vi "logic.vi"(7 "transition_queue":refnum<queue>, 8 "error in (no error)":errorcluster, 11 "data_in":T1) -> (0 "error out":errorcluster, 1 "data out":variant, 2 "change":bool, 3 "data_out":T1)   [LabVIEW 2015, in "lv-recipe-machine.lvlib"]
uses:
  lv-recipe-machine.lvlib
  _controls/recipe_data.ctl
  public/_controls/mode.ctl
  public/_controls/manual_state.ctl
  public/_controls/automatic_state.ctl
  _controls/timer.ctl
  public/_controls/recipe_step.ctl
  public/_controls/transition.ctl
  _controls/timers.ctl
  public/_controls/error.ctl
  _controls/timer_command.ctl
  _controls/automatic_vi_variant_data.ctl
  <vilib>/ptbypt/NI_PtbyPt.lvlib
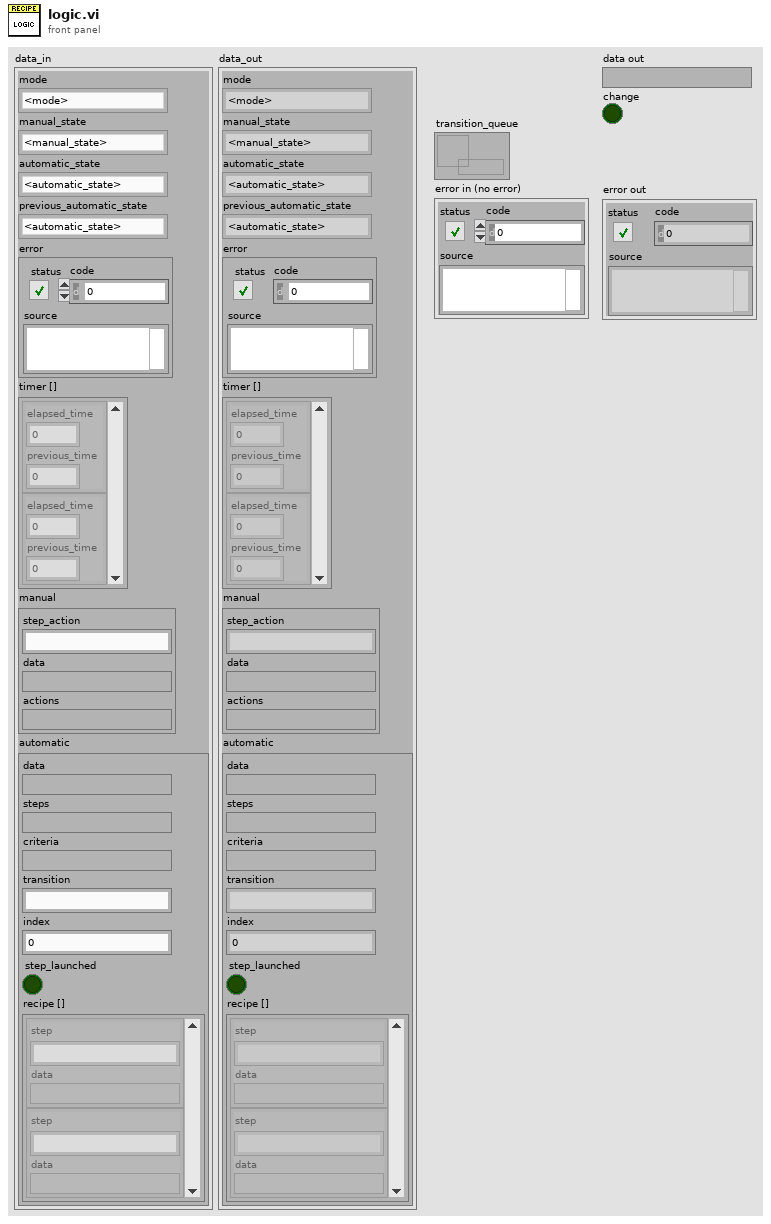
[diagram p1: front panel]
types:
  T1 = typedef "lv-recipe-machine.lvlib/recipe_data.ctl" = cluster{"mode":T2, "manual_state":T3, "automatic_state":T4, "previous_automatic_state":T4, "error":errorcluster, "timer []":T5[], "manual":cluster{"step_action":string, "data":variant, "actions":variant}, "automatic":cluster{"data":variant, "steps":variant, "criteria":variant, "transition":string, "index":i32, "step_launched":bool, "recipe []":T6[]}}
  T2 = typedef "lv-recipe-machine.lvlib/mode.ctl" = enum16{"<mode>", "manual", "automatic", "<null>"}
  T3 = typedef "lv-recipe-machine.lvlib/manual_state.ctl" = enum16{"<manual_state>", "failed", "action", "running", "idle", "<null>"}
  T4 = typedef "lv-recipe-machine.lvlib/automatic_state.ctl" = enum16{"<automatic_state>", "failed", "idle", "running", "paused", "stopped", "<null>"}
  T5 = typedef "lv-recipe-machine.lvlib/timer.ctl" = cluster{"elapsed_time":dbl, "previous_time":dbl}
  T6 = typedef "lv-recipe-machine.lvlib/recipe_step.ctl" = cluster{"step":string, "data":variant}
  T7 = typedef "lv-recipe-machine.lvlib/error.ctl" = enum16{"<error>", "bad_command", "command_queue_timeout", "stop_notifier_timeout", "die_command_timeout", "not_in_manual_mode", "not_in_automatic_mode", "not_in_automatic_idle", "not_in_automatic_running", "not_in_automatic_paused", "automatic_step_not_found", "manual_action_not_found", "automatic_not_transition_vi", "transition_step_not_found", "unsupported_vi_type", "manual_block_timeout", "<null>"}
  T8 = typedef "lv-recipe-machine.lvlib/timers.ctl" = enum16{"<timers>", "step", "recipe", "<null>"}
  T9 = typedef "lv-recipe-machine.lvlib/timer_command.ctl" = enum16{"<timer_command>", "initialize", "start", "read", "pause", "resume", "stop", "<null>"}
  T10 = typedef "lv-recipe-machine.lvlib/automatic_vi_variant_data.ctl" = cluster{"current_state":T4, "previous_state":T4, "criteria":variant, "data":variant, "recipe_data":variant, "index":i32, "step":string, "steps":variant}
  T11 = cluster{"data":variant, "steps":variant, "criteria":variant, "transition":string, "index":i32, "step_launched":bool, "recipe []":T6[]}
  T12 = cluster{"step_action":string, "data":variant, "actions":variant}
  T13 = typedef "lv-recipe-machine.lvlib/transition.ctl" = cluster{"next_index":i32, "data":variant, "recipe_data":variant, "error":errorcluster}
  T14 = cluster{"recipe_data out":variant, "error IO":errorcluster}
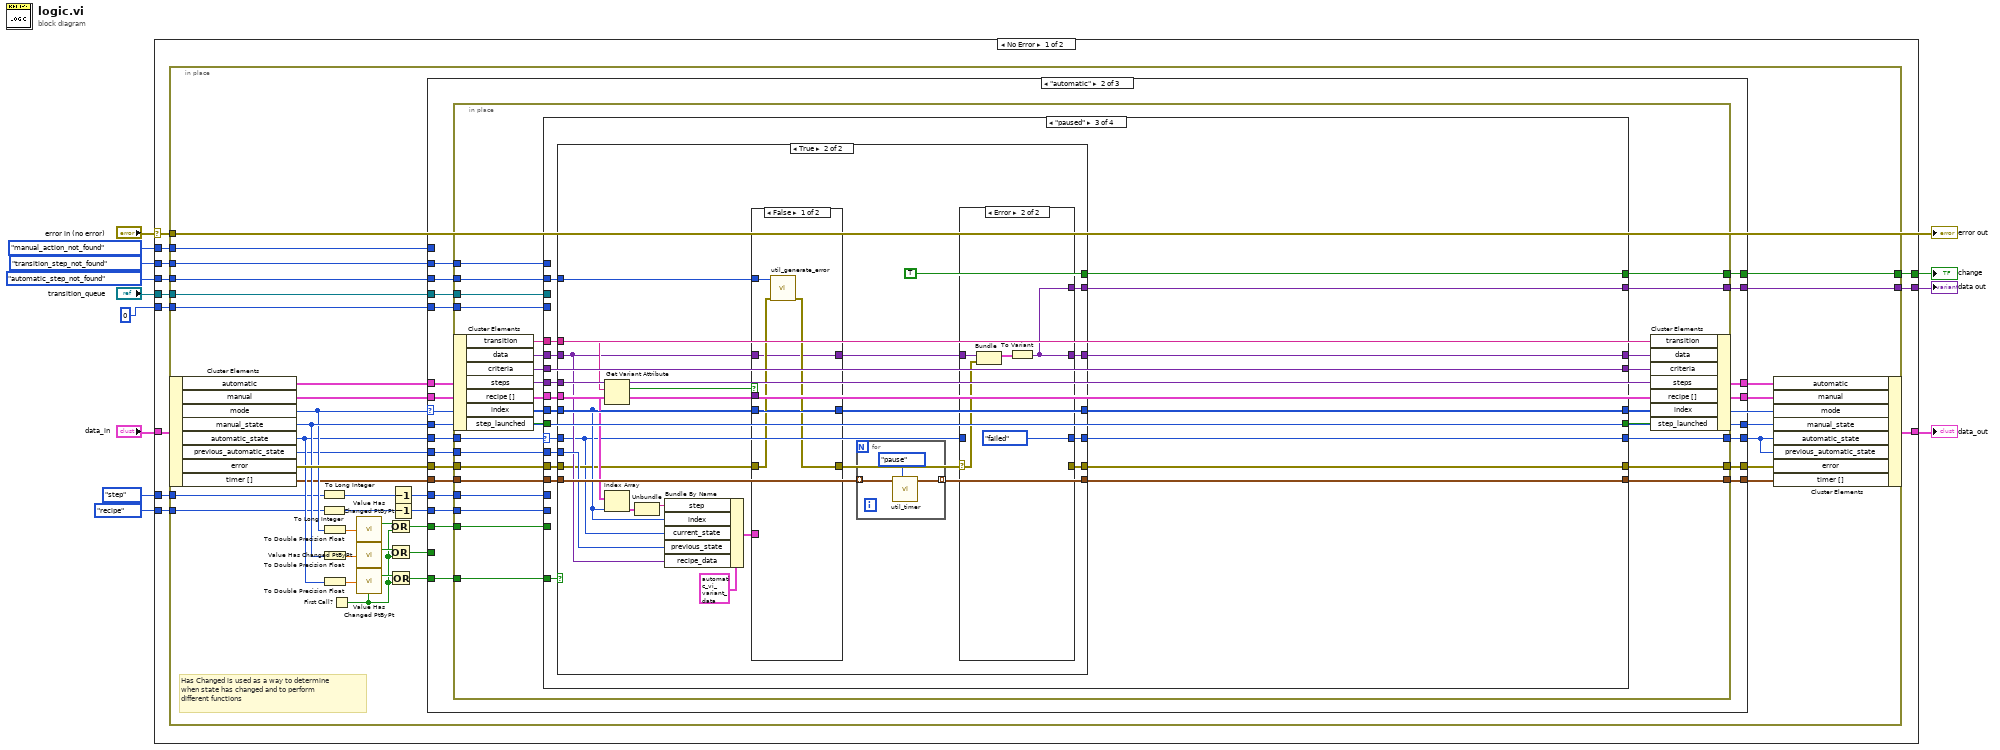
[diagram p0: block diagram]
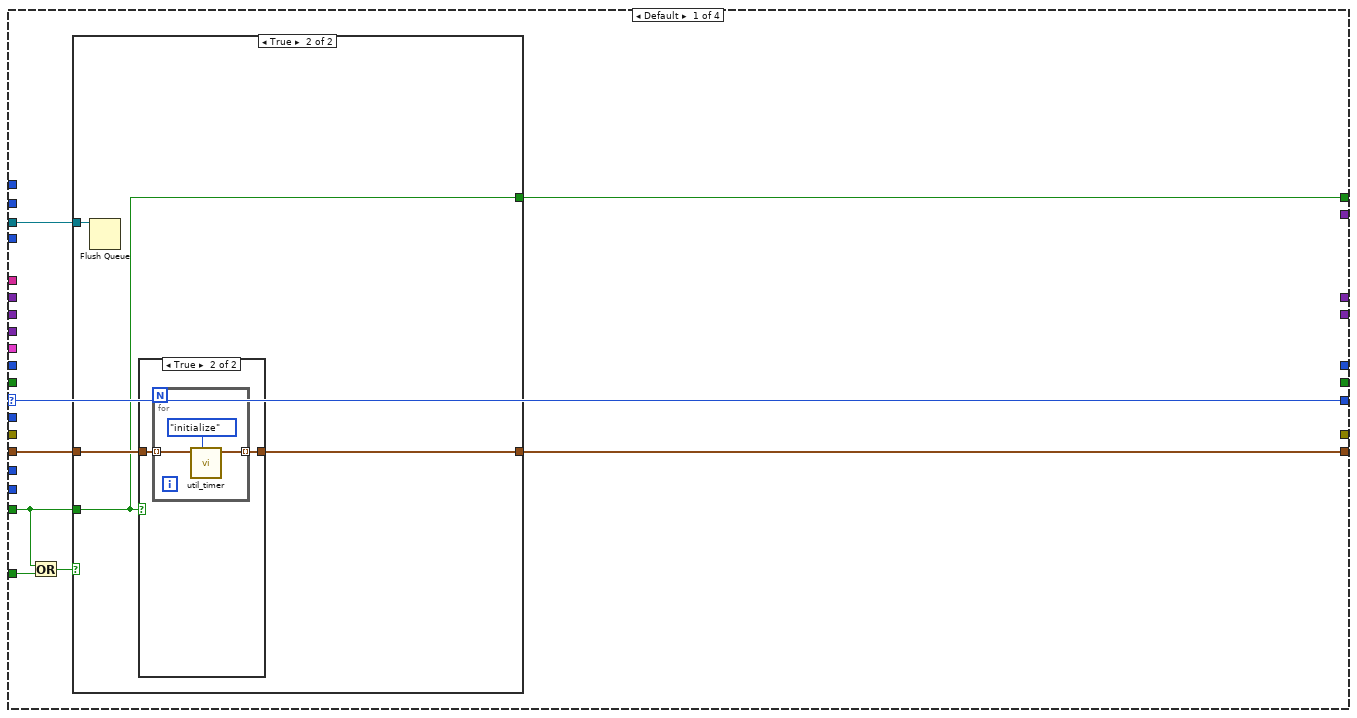
[diagram p3: hidden frame]
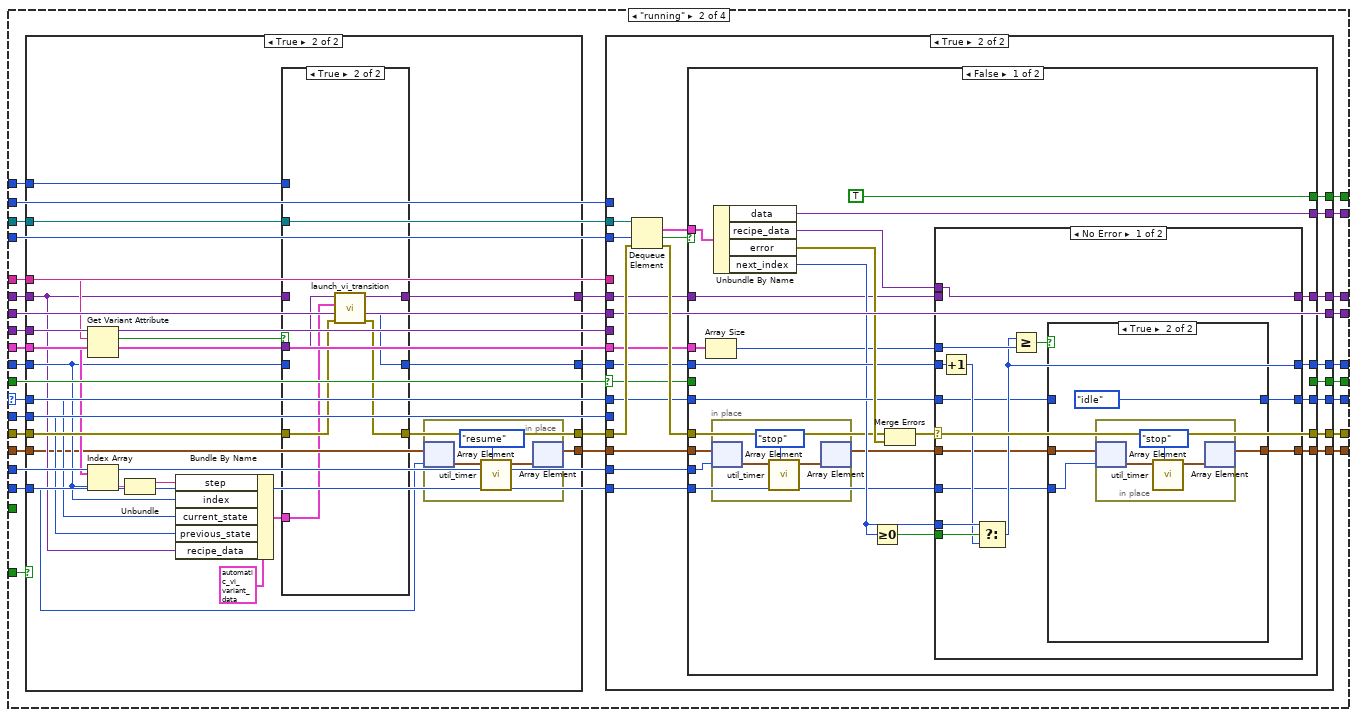
[diagram p6: hidden frame]
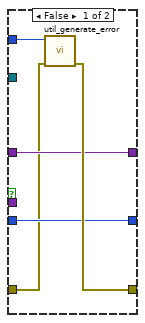
[diagram p8: hidden frame]
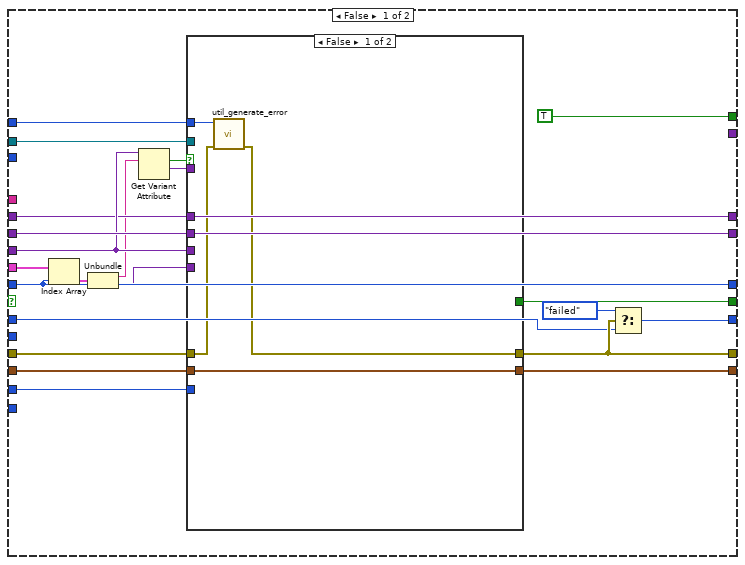
[diagram p9: hidden frame]
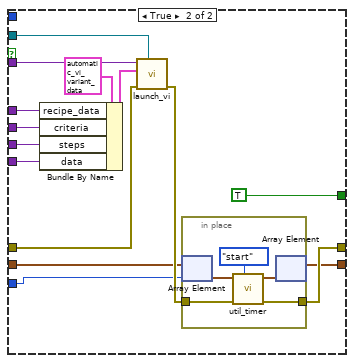
[diagram p10: hidden frame]
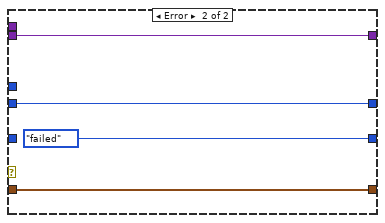
[diagram p12: hidden frame]
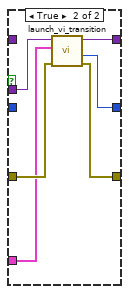
[diagram p16: hidden frame]
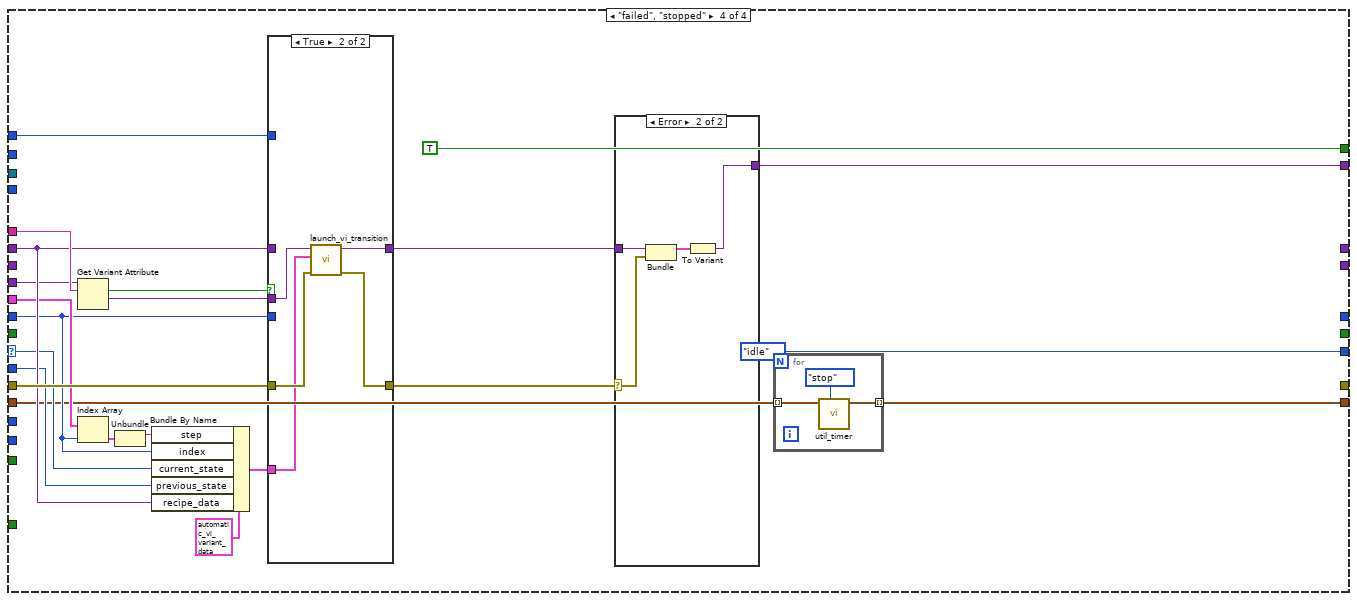
[diagram p17: hidden frame]
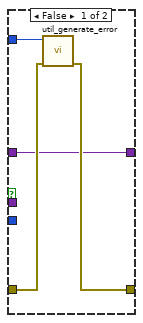
[diagram p19: hidden frame]
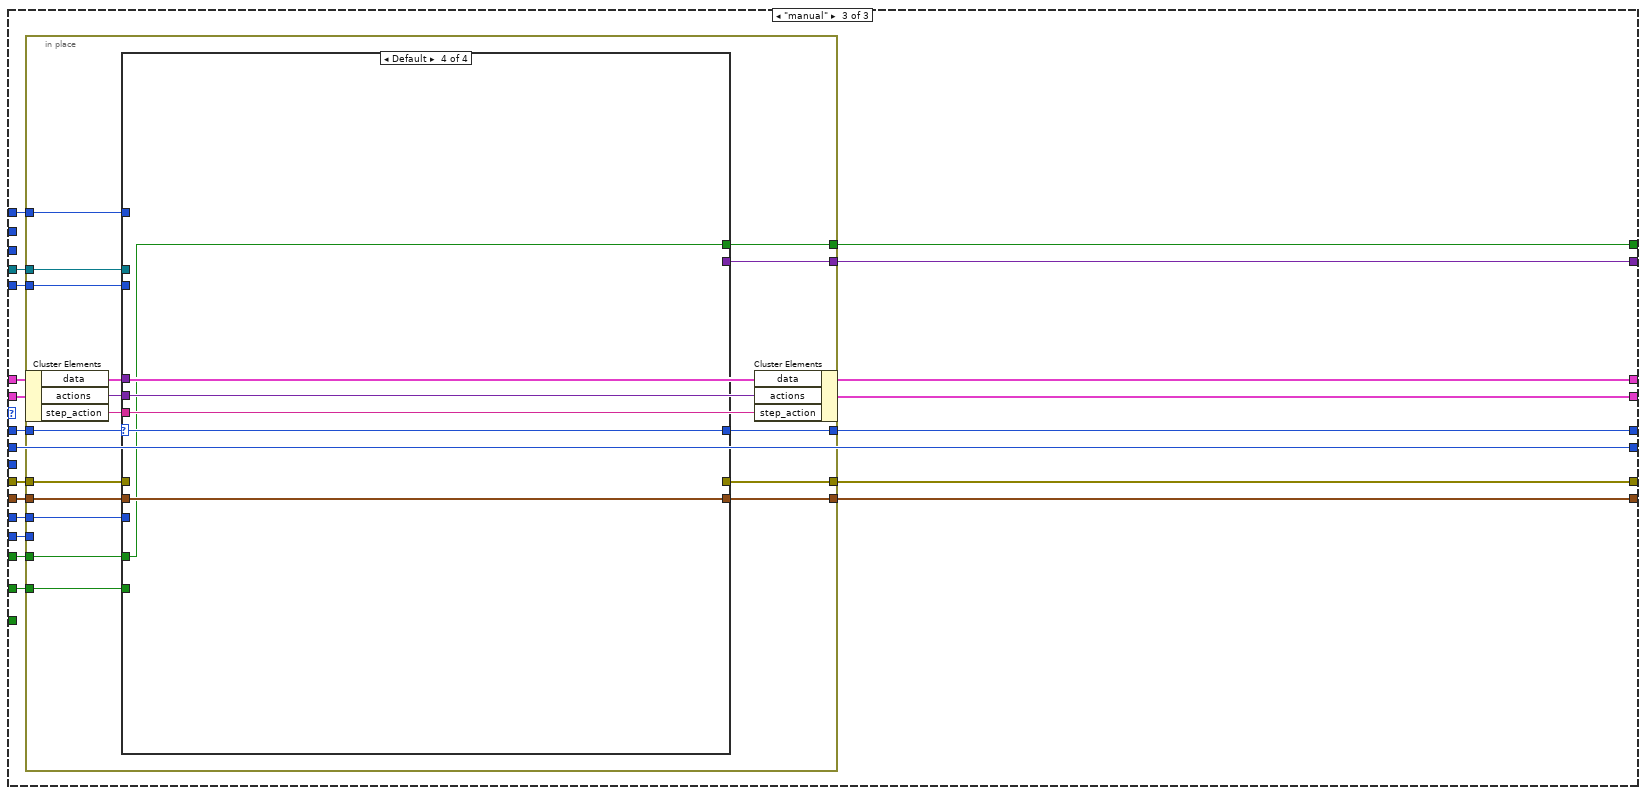
[diagram p20: hidden frame]
diagram:
  n1 = case shown="No Error" "error in (no error)" {
    selector: "error in (no error)" -> [w24 _]
    tunnel: "data_in" -> [w23 w582]
    tunnel: [w22 w582] -> w11
    tunnel: [w21 _] -> w10
    tunnel: [w20 _] -> w9
    tunnel: "transition_queue" -> [w19 _]
    tunnel: timers."step" ("timers") -> [w18 _]
    tunnel: timers."recipe" ("timers") -> [w17 _]
    tunnel: error."manual_action_not_found" ("error") -> [w16 _]
    tunnel: error."transition_step_not_found" ("error") -> [w15 _]
    tunnel: error."automatic_step_not_found" ("error") -> [w14 _]
    tunnel: 0 -> [w13 _]
    frame No Error {
      n2 = in-place {
        in-place-border: w24 -> [_]
        in-place-border: [w51] -> w21
        in-place-border: [w50] -> w20
        in-place-border: w19 -> [w41]
        in-place-border: w18 -> [w36]
        in-place-border: w17 -> [w35]
        in-place-border: w16 -> [w32]
        in-place-border: w15 -> [w31]
        in-place-border: w14 -> [w30]
        in-place-border: w13 -> [w29]
        # "Has Changed is used as a way to determine\nwhen state has changed and to perform \ndifferent functions"
        n3 = in-place-cluster #1(w23) -> ("automatic"=w46:T11, "manual"=w45:T12, "mode"=w53:T2, "manual_state"=w54:T3, "automatic_state"=w49:T4, "previous_automatic_state"=w48:T4, "error"=w61:errorcluster, "timer []"=w40:T5[])
        n4 = To Long Integer(number=w36) -> (32bit integer=w33:i32)
        n5 = To Long Integer(number=w35) -> (32bit integer=w34:i32)
        n6 = To Double Precision Float(number=w53) -> (double precision float=w60:dbl)
        n7 = To Double Precision Float(number=w54) -> (double precision float=w59:dbl)
        n8 = To Double Precision Float(number=w49) -> (double precision float=w58:dbl)
        n9 = First Call?() -> (First Call?: T/F=w25:bool)
        n10 = call <vilib>:"Value Has Changed PtByPt.vi"("input data point"=w60, "initialize"=w25) -> ("has changed"=w57:bool)  [unwired: 1 out]
        n11 = call <vilib>:"Value Has Changed PtByPt.vi"("input data point"=w59, "initialize"=w25) -> ("has changed"=w56:bool)  [unwired: 1 out]
        n12 = call <vilib>:"Value Has Changed PtByPt.vi"("input data point"=w58, "initialize"=w25) -> ("has changed"=w55:bool)  [unwired: 1 out]
        n13 = Or(x=w57, y=w25) -> (x .or. y?=w28:bool)
        n14 = Or(x=w56, y=w25) -> (x .or. y?=w27:bool)
        n15 = Or(x=w55, y=w25) -> (x .or. y?=w26:bool)
        n16 = Decrement(x=w33) -> (x-1=w38:i32)
        n17 = Decrement(x=w34) -> (x-1=w37:i32)
        n18 = case shown="\"automatic\"" w53 {
          tunnel: w54 -> [w67 w86 w461]
          tunnel: w49 -> [w66 w87 w458]
          tunnel: w28 -> [_ w71 w443]
          tunnel: w27 -> [_ _ w460]
          tunnel: w26 -> [_ w85 _]
          tunnel: [w67 w86 w459] -> w52
          tunnel: [w66 w80 w458] -> w42
          tunnel: [_ w82 w457] -> w51
          tunnel: [_ w81 w456] -> w50
          tunnel: w45 -> [w65 w88 w454]
          tunnel: w46 -> [w64 w84 w455]
          tunnel: [w64 w83 w455] -> w43
          tunnel: [w65 w88 w453] -> w44
          tunnel: w48 -> [_ w77 _]
          tunnel: w61 -> [w63 w79 w452]
          tunnel: [w63 w78 w451] -> w47
          tunnel: w41 -> [_ w76 w450]
          tunnel: w40 -> [w62 w75 w447]
          tunnel: [w62 w72 w446] -> w39
          tunnel: w38 -> [_ w74 w449]
          tunnel: w37 -> [_ w73 w448]
          tunnel: w32 -> [_ _ w445]
          tunnel: w31 -> [_ w70 _]
          tunnel: w30 -> [_ w69 _]
          tunnel: w29 -> [_ w68 w444]
          frame Default {
          }
          frame "automatic" {
            n19 = in-place {
              in-place-border: w87 -> [w94]
              in-place-border: w85 -> [w91]
              in-place-border: [w116] -> w82
              in-place-border: [w115] -> w81
              in-place-border: [w114] -> w80
              in-place-border: w79 -> [w92]
              in-place-border: [w112] -> w78
              in-place-border: w77 -> [w93]
              in-place-border: w76 -> [w101]
              in-place-border: w75 -> [w108]
              in-place-border: w74 -> [w107]
              in-place-border: w73 -> [w106]
              in-place-border: [w105] -> w72
              in-place-border: w71 -> [w89]
              in-place-border: w70 -> [w100]
              in-place-border: w69 -> [w104]
              in-place-border: w68 -> [w90]
              n20 = in-place-cluster #2(w84) -> ("transition"=w99:string, "data"=w98:variant, "criteria"=w111:variant, "steps"=w97:variant, "recipe []"=w96:T6[], "index"=w95:i32, "step_launched"=w102:bool)
              n21 = case shown="\"paused\"" w94 {
                selector: w94 -> [w124 w146 w337 w416]
                tunnel: [w119 w166 w340 TRUE] -> w116
                tunnel: [_ w165 w334 w404] -> w115
                tunnel: [w124 w164 w335 automatic_state."idle" ("automatic_state")] -> w114
                tunnel: [_ w163 w338 _] -> w113
                tunnel: [_ w162 w336 _] -> w112
                tunnel: w111 -> [_ w161 w351 _]
                tunnel: [_ w160 w351 _] -> w110
                tunnel: [_ w159 w343 _] -> w109
                tunnel: w108 -> [w121 w138 w349 w414]
                tunnel: w107 -> [_ w158 _ _]
                tunnel: w106 -> [_ w136 _ _]
                tunnel: [w120 w157 w350 w413] -> w105
                tunnel: w104 -> [_ w156 w348 _]
                tunnel: [_ w155 _ _] -> w103
                tunnel: w102 -> [_ w154 _ _]
                tunnel: w101 -> [w123 w153 _ _]
                tunnel: w100 -> [_ w152 _ w422]
                tunnel: w99 -> [_ w151 w347 w421]
                tunnel: w98 -> [_ w150 w341 w420]
                tunnel: w97 -> [_ w149 w345 w419]
                tunnel: w96 -> [_ w148 w346 w418]
                tunnel: w95 -> [_ w147 w344 w417]
                tunnel: w93 -> [_ w145 w342 w415]
                tunnel: w92 -> [_ w144 w339 w425]
                tunnel: w91 -> [w118 w140 w333 _]
                tunnel: w90 -> [_ w139 _ _]
                tunnel: w89 -> [w117 _ _ _]
                frame Default {
                  n22 = Or(x=w117, y=w118) -> (x .or. y?=w122:bool)
                  n23 = case shown="True" w122 {
                    tunnel: w123 -> [_ w129]
                    tunnel: w121 -> [w125 w128]
                    tunnel: [w125 w127] -> w120
                    tunnel: [_ w126] -> w119
                    tunnel: w117 -> [_ w126]
                    frame False {
                    }
                    frame True {
                      n24 = Flush Queue(queue=w129) -> ()  [unwired: 1 in, 3 out]
                      n25 = case shown="True" w126 {
                        tunnel: w128 -> [w130 w132]
                        tunnel: [w130 w131] -> w127
                        frame False {
                        }
                        frame True {
                          n26 = for {
                            tunnel: w132 -> [w135] mode=indexing
                            tunnel: [w134] -> w131 mode=indexing
                            n27 = call "util_timer.vi"("timer_command"=timer_command."initialize", "timer in"=w135) -> ("timer out"=w134:T5)  [unwired: 7 in, 2 out]
                          }
                        }
                      }
                    }
                  }
                }
                frame "running" {
                  n28 = case shown="True" w140 {
                    tunnel: [w168 w191] -> w143
                    tunnel: w150 -> [w169 w177]
                    tunnel: w146 -> [_ w180]
                    tunnel: w145 -> [_ w179]
                    tunnel: w149 -> [_ w190]
                    tunnel: [w169 w188] -> w141
                    tunnel: w147 -> [w170 w182]
                    tunnel: [w170 w187] -> w142
                    tunnel: w151 -> [_ w189]
                    tunnel: w148 -> [_ w183]
                    tunnel: w153 -> [_ w176]
                    tunnel: w152 -> [_ w174]
                    tunnel: w144 -> [w168 w192]
                    tunnel: w138 -> [w167 w172]
                    tunnel: [w167 w173] -> w137
                    tunnel: w136 -> [_ w171]
                    frame False {
                    }
                    frame True {
                      n29 = Get Variant Attribute(Variant=w190, name=w189) -> (found=w186:bool, value=w175:variant)  [unwired: 2 in, 2 out]
                      n30 = Index Array(array=w183, index=w182) -> (element=w181:T6)
                      n31 = Unbundle(w181) -> ("step"=w178:string)  [unwired: 1 out]
                      n32 = Bundle By Name(cluster=T10 {"current_state"=enum."<automatic_state>", "previous_state"=enum."<automatic_state>", "criteria"=variant, "data"=variant, "recipe_data"=variant, "index"=0, "step"="", "steps"=variant} ("data"), "step"=w178, "index"=w182, "current_state"=w180, "previous_state"=w179, "recipe_data"=w177) -> (w184:T10)
                      n33 = case shown="True" w186 {
                        tunnel: [w200 w205] -> w191
                        tunnel: w175 -> [_ w204]
                        tunnel: w177 -> [w199 _]
                        tunnel: [w199 w201] -> w188
                        tunnel: w182 -> [w198 _]
                        tunnel: [w198 w203] -> w187
                        tunnel: w184 -> [_ w202]
                        tunnel: w176 -> [_ _]
                        tunnel: w174 -> [w197 _]
                        tunnel: w192 -> [w196 w206]
                        frame False {
                          n34 = call "util_generate_error.vi"("error in (no error)"=w196, "error"=w197) -> ("error out"=w200:errorcluster)  [unwired: 9 in]
                        }
                        frame True {
                          n35 = call "launch_vi_transition.vi"("error in (no error)"=w206, "data"=w202, "vi_reference"=w204) -> ("error out"=w205:errorcluster, "index out"=w203:i32, "recipe_data out"=w201:variant)  [unwired: 6 in]
                        }
                      }
                      n36 = in-place {
                        n37 = in-place-array #3(w172, w171) -> (w194:T5)
                        n38 = call "util_timer.vi"("timer_command"=timer_command."resume", "timer in"=w194) -> ("timer out"=w193:T5)  [unwired: 7 in, 2 out]
                        n39 = in-place-array #3(w193) -> (w173:T5[])  [unwired: 1 out]
                      }
                    }
                  }
                  n40 = case shown="True" w154 {
                    selector: w154 -> [_ w254]
                    tunnel: w146 -> [w224 w273]
                    tunnel: w149 -> [w223 _]
                    tunnel: w142 -> [w213 w272]
                    tunnel: w148 -> [w222 w271]
                    tunnel: [TRUE w270] -> w166
                    tunnel: [_ w269] -> w165
                    tunnel: [w227 w268] -> w164
                    tunnel: w141 -> [w215 w267]
                    tunnel: [w215 w266] -> w163
                    tunnel: w143 -> [w214 w275]
                    tunnel: [w226 w265] -> w162
                    tunnel: w161 -> [w225 w264]
                    tunnel: [w225 w264] -> w160
                    tunnel: w151 -> [_ _]
                    tunnel: w145 -> [_ _]
                    tunnel: [w213 w263] -> w159
                    tunnel: w153 -> [w221 w262]
                    tunnel: w137 -> [w220 w261]
                    tunnel: w158 -> [w219 w259]
                    tunnel: w136 -> [_ w258]
                    tunnel: [w218 w260] -> w157
                    tunnel: w156 -> [w217 _]
                    tunnel: [w216 w253] -> w155
                    tunnel: w139 -> [_ w255]
                    frame False {
                      n41 = Index Array(array=w222, index=w213) -> (element=w209:T6)
                      n42 = Unbundle(w209) -> ("step"=w208:string, "data"=w207:variant)
                      n43 = Get Variant Attribute(Variant=w223, name=w208) -> (found=w211:bool, value=w212:variant)  [unwired: 2 in, 2 out]
                      n44 = case shown="False" w211 {
                        tunnel: w212 -> [_ w234]
                        tunnel: w207 -> [_ w241]
                        tunnel: w214 -> [w232 w246]
                        tunnel: [w231 w236] -> w226
                        tunnel: w225 -> [_ w243]
                        tunnel: w215 -> [_ w242]
                        tunnel: w223 -> [_ w240]
                        tunnel: w221 -> [_ w239]
                        tunnel: w220 -> [w230 w238]
                        tunnel: w219 -> [_ w237]
                        tunnel: [w230 w235] -> w218
                        tunnel: w217 -> [w229 _]
                        tunnel: [_ TRUE] -> w216
                        frame False {
                          n45 = call "util_generate_error.vi"("error in (no error)"=w232, "error"=w229) -> ("error out"=w231:errorcluster)  [unwired: 9 in]
                        }
                        frame True {
                          n46 = Bundle By Name(cluster=T10 {"current_state"=enum."<automatic_state>", "previous_state"=enum."<automatic_state>", "criteria"=variant, "data"=variant, "recipe_data"=variant, "index"=0, "step"="", "steps"=variant} ("data"), "recipe_data"=w242, "criteria"=w243, "steps"=w240, "data"=w241) -> (w245:T10)
                          n47 = call "launch_vi.vi"("transition_queue"=w239, "error in (no error)"=w246, "data"=w245, "vi_reference"=w234) -> ("error out"=w247:errorcluster)  [unwired: 7 in]
                          n48 = in-place {
                            in-place-border: w247 -> [w249]
                            in-place-border: [w248] -> w236
                            n49 = in-place-array #4(w238, w237) -> (w251:T5)
                            n50 = call "util_timer.vi"("timer_command"=timer_command."start", "error in (no error)"=w249, "timer in"=w251) -> ("error out"=w248:errorcluster, "timer out"=w250:T5)  [unwired: 6 in, 1 out]
                            n51 = in-place-array #4(w250) -> (w235:T5[])  [unwired: 1 out]
                          }
                        }
                      }
                      n52 = Select(t=automatic_state."failed", s=w226, f=w224) -> (s? t:f=w227:T4)
                    }
                    frame True {
                      n53 = Dequeue Element(queue=w262, timeout in ms (-1)=w255, error in (no error)=w275) -> (element=w257:T13, timed out?=w256:bool, error out=w274:errorcluster)  [unwired: 1 out]
                      n54 = case shown="False" w256 {
                        tunnel: [TRUE _] -> w270
                        tunnel: [w294 _] -> w269
                        tunnel: w273 -> [w291 w332]
                        tunnel: [w293 w332] -> w268
                        tunnel: w272 -> [w292 w329]
                        tunnel: w271 -> [w279 _]
                        tunnel: w257 -> [w295 _]
                        tunnel: w267 -> [w287 w331]
                        tunnel: [w286 w331] -> w266
                        tunnel: w274 -> [w277 w330]
                        tunnel: [w276 w330] -> w265
                        tunnel: [w288 w329] -> w263
                        tunnel: w261 -> [w284 w328]
                        tunnel: w259 -> [w283 _]
                        tunnel: [w280 w328] -> w260
                        tunnel: w258 -> [w281 _]
                        tunnel: w254 -> [_ w327]
                        tunnel: [_ w327] -> w253
                        frame False {
                          n55 = Array Size(array=w279) -> (size(s)=w278:i32)
                          n56 = in-place {
                            n57 = in-place-array #5(w284, w283) -> (w299:T5)
                            n58 = call "util_timer.vi"("timer_command"=timer_command."stop", "timer in"=w299) -> ("timer out"=w298:T5)  [unwired: 7 in, 2 out]
                            n59 = in-place-array #5(w298) -> (w282:T5[])  [unwired: 1 out]
                          }
                          n60 = Unbundle By Name(w295) -> ("data"=w294:variant, "recipe_data"=w285:variant, "error"=w297:errorcluster, "next_index"=w290:i32)
                          n61 = Greater Or Equal To 0?(x=w290) -> (x >= 0?=w289:bool)
                          n62 = Merge Errors(w277, w297) -> (w276:errorcluster)
                          n63 = case shown="No Error" w276 {
                            tunnel: [w304 automatic_state."failed" ("t")] -> w293
                            tunnel: w292 -> [w312 w325]
                            tunnel: w291 -> [w305 _]
                            tunnel: w278 -> [w313 _]
                            tunnel: [w308 w325] -> w288
                            tunnel: w290 -> [w310 _]
                            tunnel: w289 -> [w311 _]
                            tunnel: w287 -> [_ w324]
                            tunnel: [w307 w324] -> w286
                            tunnel: w285 -> [w307 _]
                            tunnel: w282 -> [w303 w323]
                            tunnel: w281 -> [w302 _]
                            tunnel: [w301 w323] -> w280
                            frame No Error {
                              n64 = Increment(x=w312) -> (x+1=w309:i32)
                              n65 = Select(t=w310, s=w311, f=w309) -> (s? t:f=w308:i32)
                              n66 = Greater Or Equal?(x=w308, y=w313) -> (x >= y?=w306:bool)
                              n67 = case shown="True" w306 {
                                tunnel: w305 -> [w315 _]
                                tunnel: [w315 automatic_state."idle" ("t")] -> w304
                                tunnel: w303 -> [w314 w318]
                                tunnel: w302 -> [_ w317]
                                tunnel: [w314 w316] -> w301
                                frame False {
                                }
                                frame True {
                                n68 = in-place {
                                n69 = in-place-array #6(w318, w317) -> (w321:T5)
                                n70 = call "util_timer.vi"("timer_command"=timer_command."stop", "timer in"=w321) -> ("timer out"=w320:T5)  [unwired: 7 in, 2 out]
                                n71 = in-place-array #6(w320) -> (w316:T5[])  [unwired: 1 out]
                                }
                                }
                              }
                            }
                            frame Error {
                            }
                          }
                        }
                        frame True {
                        }
                      }
                    }
                  }
                }
                frame "paused" {
                  n72 = case shown="True" w333 {
                    tunnel: [w354 w374] -> w350
                    tunnel: w349 -> [w354 w373]
                    tunnel: w348 -> [_ w372]
                    tunnel: w347 -> [_ w371]
                    tunnel: w346 -> [_ w370]
                    tunnel: w345 -> [_ w369]
                    tunnel: w344 -> [w352 w368]
                    tunnel: [w352 w367] -> w343
                    tunnel: w342 -> [_ w366]
                    tunnel: w341 -> [w356 w365]
                    tunnel: [_ TRUE] -> w340
                    tunnel: w339 -> [w355 w363]
                    tunnel: [w356 w361] -> w338
                    tunnel: w337 -> [w353 w360]
                    tunnel: [w355 w359] -> w336
                    tunnel: [w353 w358] -> w335
                    tunnel: [_ w357] -> w334
                    frame False {
                    }
                    frame True {
                      n73 = Get Variant Attribute(Variant=w369, name=w371) -> (found=w380:bool, value=w375:variant)  [unwired: 2 in, 2 out]
                      n74 = Index Array(array=w370, index=w368) -> (element=w377:T6)
                      n75 = Unbundle(w377) -> ("step"=w376:string)  [unwired: 1 out]
                      n76 = Bundle By Name(cluster=T10 {"current_state"=enum."<automatic_state>", "previous_state"=enum."<automatic_state>", "criteria"=variant, "data"=variant, "recipe_data"=variant, "index"=0, "step"="", "steps"=variant} ("data"), "step"=w376, "index"=w368, "current_state"=w360, "previous_state"=w366, "recipe_data"=w365) -> (w378:T10)
                      n77 = case shown="False" w380 {
                        tunnel: [w394 w399] -> w362
                        tunnel: w375 -> [_ w398]
                        tunnel: w365 -> [w392 _]
                        tunnel: [w392 w396] -> w381
                        tunnel: w368 -> [w390 _]
                        tunnel: w378 -> [_ w397]
                        tunnel: w372 -> [w391 _]
                        tunnel: [w390 w395] -> w367
                        tunnel: w363 -> [w393 w400]
                        frame False {
                          n78 = call "util_generate_error.vi"("error in (no error)"=w393, "error"=w391) -> ("error out"=w394:errorcluster)  [unwired: 9 in]
                        }
                        frame True {
                          n79 = call "launch_vi_transition.vi"("error in (no error)"=w400, "data"=w397, "vi_reference"=w398) -> ("error out"=w399:errorcluster, "index out"=w395:i32, "recipe_data out"=w396:variant)  [unwired: 6 in]
                        }
                      }
                      n80 = for {
                        tunnel: w373 -> [w403] mode=indexing
                        tunnel: [w402] -> w374 mode=indexing
                        n81 = call "util_timer.vi"("timer_command"=timer_command."pause", "timer in"=w403) -> ("timer out"=w402:T5)  [unwired: 7 in, 2 out]
                      }
                      n82 = case shown="Error" w362 {
                        selector: w362 -> [w384 w387]
                        tunnel: w381 -> [w382 w389]
                        tunnel: [w382 w386] -> w361
                        tunnel: w360 -> [w383 _]
                        tunnel: [w384 _] -> w359
                        tunnel: [w383 automatic_state."failed" ("automatic_state")] -> w358
                        tunnel: [_ w386] -> w357
                        frame No Error {
                        }
                        frame Error {
                          n83 = Bundle("recipe_data out"=w389, "error IO"=w387) -> (w388:T14)  [unwired: 1 in]
                          n84 = To Variant(anything=w388) -> (Variant=w386:variant)
                        }
                      }
                    }
                  }
                }
                frame "failed", "stopped" {
                  n85 = Get Variant Attribute(Variant=w419, name=w421) -> (found=w412:bool, value=w407:variant)  [unwired: 2 in, 2 out]
                  n86 = Index Array(array=w418, index=w417) -> (element=w409:T6)
                  n87 = Unbundle(w409) -> ("step"=w408:string)  [unwired: 1 out]
                  n88 = Bundle By Name(cluster=T10 {"current_state"=enum."<automatic_state>", "previous_state"=enum."<automatic_state>", "criteria"=variant, "data"=variant, "recipe_data"=variant, "index"=0, "step"="", "steps"=variant} ("data"), "step"=w408, "index"=w417, "current_state"=w416, "previous_state"=w415, "recipe_data"=w420) -> (w410:T10)
                  n89 = case shown="True" w412 {
                    tunnel: [w433 w438] -> w405
                    tunnel: w407 -> [_ w437]
                    tunnel: w420 -> [w432 _]
                    tunnel: [w432 w435] -> w406
                    tunnel: w417 -> [_ _]
                    tunnel: w410 -> [_ w436]
                    tunnel: w422 -> [w431 _]
                    tunnel: w425 -> [w434 w439]
                    frame False {
                      n90 = call "util_generate_error.vi"("error in (no error)"=w434, "error"=w431) -> ("error out"=w433:errorcluster)  [unwired: 9 in]
                    }
                    frame True {
                      n91 = call "launch_vi_transition.vi"("error in (no error)"=w439, "data"=w436, "vi_reference"=w437) -> ("error out"=w438:errorcluster, "recipe_data out"=w435:variant)  [unwired: 6 in, 1 out]
                    }
                  }
                  n92 = case shown="Error" w405 {
                    selector: w405 -> [_ w428]
                    tunnel: w406 -> [w426 w429]
                    tunnel: [w426 w427] -> w404
                    frame No Error {
                    }
                    frame Error {
                      n93 = Bundle("recipe_data out"=w429, "error IO"=w428) -> (w430:T14)  [unwired: 1 in]
                      n94 = To Variant(anything=w430) -> (Variant=w427:variant)
                    }
                  }
                  n95 = for {
                    tunnel: w414 -> [w442] mode=indexing
                    tunnel: [w441] -> w413 mode=indexing
                    n96 = call "util_timer.vi"("timer_command"=timer_command."stop", "timer in"=w442) -> ("timer out"=w441:T5)  [unwired: 7 in, 2 out]
                  }
                }
              }
              n97 = in-place-cluster #2("transition"=w99, "data"=w113, "criteria"=w110, "steps"=w97, "recipe []"=w96, "index"=w109, "step_launched"=w103) -> (w83:T11)
            }
          }
          frame "manual" {
            n98 = in-place {
              in-place-border: w461 -> [w478]
              in-place-border: w460 -> [w477]
              in-place-border: [w476] -> w459
              in-place-border: [w475] -> w457
              in-place-border: [w474] -> w456
              in-place-border: w452 -> [w470]
              in-place-border: [w469] -> w451
              in-place-border: w450 -> [w468]
              in-place-border: w449 -> [w467]
              in-place-border: w448 -> [_]
              in-place-border: w447 -> [w466]
              in-place-border: [w465] -> w446
              in-place-border: w445 -> [w464]
              in-place-border: w444 -> [w463]
              in-place-border: w443 -> [w462]
              n99 = in-place-cluster #7(w454) -> ("data"=w473:variant, "actions"=w472:variant, "step_action"=w471:string)
              n100 = case shown="Default" w478 {
                selector: w478 -> [w489 w545 _ w581]
                tunnel: w471 -> [w486 _ _ _]
                tunnel: [w492 w546 manual_state."idle" ("manual_state") w581] -> w476
                tunnel: [w491 w544 TRUE w579] -> w475
                tunnel: [_ w543 w573 _] -> w474
                tunnel: w477 -> [w490 _ _ _]
                tunnel: w472 -> [w488 _ _ _]
                tunnel: w473 -> [w487 _ w569 _]
                tunnel: [w485 w542 _ _] -> w469
                tunnel: w470 -> [w484 w535 w568 _]
                tunnel: w468 -> [w483 w539 _ _]
                tunnel: w467 -> [w482 w537 w571 _]
                tunnel: w466 -> [w481 w538 w572 w580]
                tunnel: [w480 w536 w570 w580] -> w465
                tunnel: w464 -> [w479 _ _ _]
                tunnel: w463 -> [_ w533 _ _]
                tunnel: w462 -> [_ _ _ w579]
                frame "action" {
                  n101 = case shown="True" w490 {
                    tunnel: [w495 w507] -> w492
                    tunnel: [_ TRUE] -> w491
                    tunnel: w486 -> [_ w505]
                    tunnel: w489 -> [w495 _]
                    tunnel: w488 -> [_ w504]
                    tunnel: w487 -> [_ w503]
                    tunnel: [w494 w502] -> w485
                    tunnel: w484 -> [w494 w497]
                    tunnel: w483 -> [_ w501]
                    tunnel: w482 -> [_ w500]
                    tunnel: w481 -> [w493 w499]
                    tunnel: [w493 w498] -> w480
                    tunnel: w479 -> [_ w496]
                    frame False {
                    }
                    frame True {
                      n102 = Get Variant Attribute(Variant=w504, name=w505) -> (found=w510:bool, value=w511:variant)  [unwired: 2 in, 2 out]
                      n103 = case shown="True" w510 {
                        tunnel: w511 -> [_ w517]
                        tunnel: [w515 w525] -> w502
                        tunnel: w503 -> [_ w522]
                        tunnel: w501 -> [_ w521]
                        tunnel: w500 -> [_ w518]
                        tunnel: w499 -> [w513 w520]
                        tunnel: [w513 w519] -> w498
                        tunnel: w497 -> [w514 w516]
                        tunnel: w496 -> [w512 _]
                        frame False {
                          n104 = call "util_generate_error.vi"("error in (no error)"=w514, "error"=w512) -> ("error out"=w515:errorcluster)  [unwired: 9 in]
                        }
                        frame True {
                          n105 = Bundle By Name(cluster=T10 {"current_state"=enum."<automatic_state>", "previous_state"=enum."<automatic_state>", "criteria"=variant, "data"=variant, "recipe_data"=variant, "index"=0, "step"="", "steps"=variant} ("data"), "data"=w522) -> (w523:T10)
                          n106 = call "launch_vi.vi"("transition_queue"=w521, "error in (no error)"=w516, "data"=w523, "vi_reference"=w517) -> ("error out"=w526:errorcluster)  [unwired: 7 in]
                          n107 = in-place {
                            in-place-border: w526 -> [w530]
                            in-place-border: [w529] -> w525
                            in-place-border: [w527] -> _
                            n108 = in-place-array #8(w520, w518) -> (w532:T5)
                            n109 = call "util_timer.vi"("timer_command"=timer_command."start", "error in (no error)"=w530, "timer in"=w532) -> ("error out"=w529:errorcluster, "elapsed_time"=w527:dbl, "timer out"=w531:T5)  [unwired: 6 in]
                            n110 = in-place-array #8(w531) -> (w519:T5[])  [unwired: 1 out]
                          }
                        }
                      }
                      n111 = Select(t=manual_state."failed" ("manual_state"), s=w502, f=manual_state."running" ("manual_state")) -> (s? t:f=w507:T3)
                    }
                  }
                }
                frame "running" {
                  n112 = Dequeue Element(queue=w539, timeout in ms (-1)=w533, error in (no error)=w535) -> (element=w541:T13, timed out?=w540:bool, error out=w534:errorcluster)  [unwired: 1 out]
                  n113 = case shown="False" w540 {
                    tunnel: w541 -> [w557 _]
                    tunnel: [w556 w566] -> w546
                    tunnel: w545 -> [_ w566]
                    tunnel: [TRUE _] -> w544
                    tunnel: [w552 _] -> w543
                    tunnel: [w548 w565] -> w542
                    tunnel: w534 -> [_ w565]
                    tunnel: w538 -> [w551 w564]
                    tunnel: w537 -> [w550 _]
                    tunnel: [w547 w564] -> w536
                    frame False {
                      n114 = Unbundle By Name(w557) -> ("data"=w552:variant, "error"=w549:errorcluster)
                      n115 = in-place {
                        in-place-border: w549 -> [w560]
                        in-place-border: [w559] -> w548
                        in-place-border: [w558] -> _
                        n116 = in-place-array #9(w551, w550) -> (w563:T5)
                        n117 = call "util_timer.vi"("timer_command"=timer_command."stop", "error in (no error)"=w560, "timer in"=w563) -> ("error out"=w559:errorcluster, "elapsed_time"=w558:dbl, "timer out"=w562:T5)  [unwired: 6 in]
                        n118 = in-place-array #9(w562) -> (w547:T5[])  [unwired: 1 out]
                      }
                      n119 = Select(t=manual_state."failed" ("manual_state"), s=w548, f=manual_state."idle" ("manual_state")) -> (s? t:f=w556:T3)
                    }
                    frame True {
                    }
                  }
                }
                frame "failed" {
                  n120 = in-place {
                    n121 = in-place-array #10(w572, w571) -> (w577:T5)
                    n122 = call "util_timer.vi"("timer_command"=timer_command."stop", "timer in"=w577) -> ("timer out"=w576:T5)  [unwired: 7 in, 2 out]
                    n123 = in-place-array #10(w576) -> (w570:T5[])  [unwired: 1 out]
                  }
                  n124 = Bundle("data"=w569, "error"=w568) -> (w567:cluster{"data":variant, "error":errorcluster})  [unwired: 1 in]
                  n125 = To Variant(anything=w567) -> (Variant=w573:variant)
                }
                frame Default {
                }
              }
              n126 = in-place-cluster #7("data"=w473, "actions"=w472, "step_action"=w471) -> (w453:T12)
            }
          }
        }
        n127 = in-place-cluster #1("automatic"=w43, "manual"=w44, "mode"=w53, "manual_state"=w52, "automatic_state"=w42, "previous_automatic_state"=w42, "error"=w47, "timer []"=w39) -> (w22:T1)
      }
    }
    frame Error {
    }
  }
  "data_out" <- w11
  "change" <- w10
  "data out" <- w9
  "error out" <- "error in (no error)"
